vi "Init Device.vi"(8 "error in (no error)":errorcluster, 11 "Ti2 in":refnum<class "Ti2.lvclass">) -> (0 "error out":errorcluster, 3 "Ti2 out":refnum<class "Ti2.lvclass">)   [LabVIEW 2016, in "Ti2.lvlib" / "Ti2.lvclass"]
uses:
  Ti2.lvclass
  Device/Device.lvclass
  ti2lv/ti2lv.lvlib
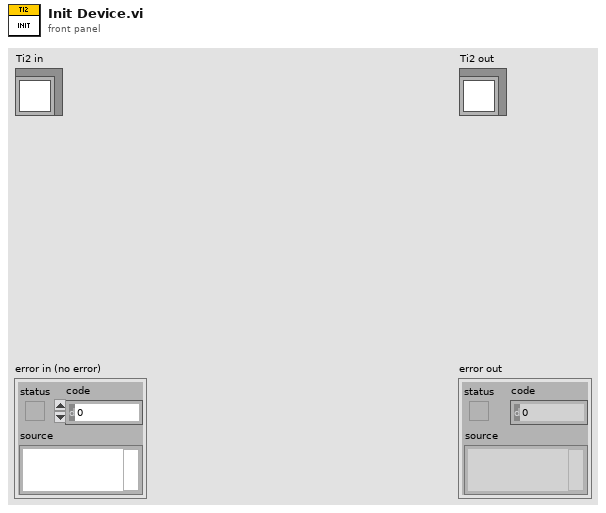
[diagram p1: front panel]
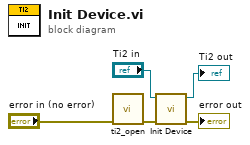
[diagram p0: block diagram]
diagram:
  n1 = call "ti2_open.vi"("error in (no error)"="error in (no error)") -> ("error out"=w1:errorcluster)  [unwired: 10 in]
  n2 = call-parent "Init Device.vi"("error in (no error)"=w1, "Device in"="Ti2 in") -> ("error out"=→"error out":errorcluster, "Device out"=→"Ti2 out":refnum<class "Ti2.lvclass">)  [unwired: 8 in]
